vi "Event Programing.vi"() -> ()   [LabVIEW 2018]
panel:
  out "Count":i32
  in  "이벤트 타임 아웃":i32=-1
  in  "정지 버튼":bool
  in  "버튼":cluster{"버튼1":bool, "버튼2":bool, "버튼3":bool}
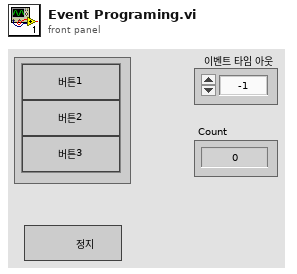
[diagram p1: front panel]
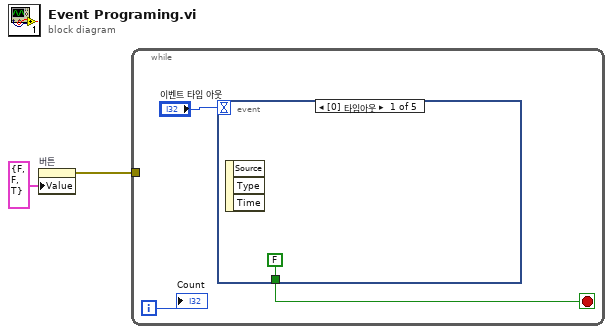
[diagram p0: block diagram]
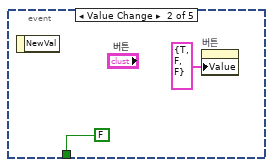
[diagram p2: hidden frame]
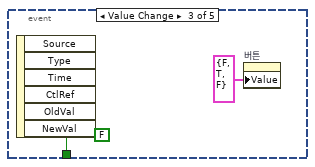
[diagram p3: hidden frame]
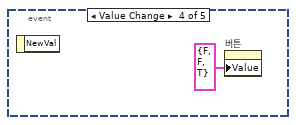
[diagram p4: hidden frame]
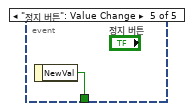
[diagram p5: hidden frame]
diagram:
  n1 = property on="버튼" class="Clust (엄격한)"("Value"=cluster{"버튼1":bool, "버튼2":bool, "버튼3":bool} {"버튼1"=FALSE, "버튼2"=FALSE, "버튼3"=TRUE} ("버튼")) -> (error out=w1:errorcluster)  [unwired: 2 in, 1 out]
  n2 = while {
    tunnel: w1 -> [_]
    i -> [w3]
    stop <- w5 stop-if-true
    n3 = event shown="[0] 타임아웃" {
      selector: _ -> [_ _ _ _ _]
      dyn-events: _ -> [_ _ _ _ _]
      timeout: "이벤트 타임 아웃" -> [_ _ _ _ _]
      tunnel: [FALSE ("NewVal") FALSE ("NewVal") FALSE ("NewVal") _ w12] -> w5
      event Timeout {
        n4 = event-data() -> ()  [unwired: 1 in, 3 out]
      }
      event "버튼.버튼1": Value Change {
        n5 = event-data() -> ()  [unwired: 1 in, 1 out]
        n6 = property on="버튼" class="Clust (엄격한)"("Value"=cluster{"버튼1":bool, "버튼2":bool, "버튼3":bool} {"버튼1"=TRUE, "버튼2"=FALSE, "버튼3"=FALSE} ("버튼")) -> ()  [unwired: 2 in, 2 out]
      }
      event "버튼.버튼2": Value Change {
        n7 = event-data() -> ()  [unwired: 1 in, 6 out]
        n8 = property on="버튼" class="Clust (엄격한)"("Value"=cluster{"버튼1":bool, "버튼2":bool, "버튼3":bool} {"버튼1"=FALSE, "버튼2"=TRUE, "버튼3"=FALSE} ("버튼")) -> ()  [unwired: 2 in, 2 out]
      }
      event "버튼.버튼3": Value Change {
        n9 = event-data() -> ()  [unwired: 1 in, 1 out]
        n10 = property on="버튼" class="Clust (엄격한)"("Value"=cluster{"버튼1":bool, "버튼2":bool, "버튼3":bool} {"버튼1"=FALSE, "버튼2"=FALSE, "버튼3"=TRUE} ("버튼")) -> ()  [unwired: 2 in, 2 out]
      }
      event "정지 버튼": Value Change {
        n11 = event-data() -> ("NewVal"=w12:bool)  [unwired: 1 in]
      }
    }
    "Count" <- w3
  }
